vi "beginPrepareKickoffEnemyPlayVSS.vi"(8 "error in (no error)":errorcluster, 10 "Game in":refnum<class "Game.lvclass">, 11 "PrepareKickoffEnemyPlayVSS in":refnum<class "PrepareKickoffEnemyPlayVSS.lvclass">) -> (0 "error out":errorcluster, 2 "Boolean":bool, 3 "PrepareKickoffEnemyPlayVSS out":refnum<class "PrepareKickoffEnemyPlayVSS.lvclass">)   [LabVIEW 2020, in "PrepareKickoffEnemyPlayVSS.lvclass"]
uses:
  PrepareKickoffEnemyPlayVSS.lvclass
  Game_class/Game.lvclass
  Game_class/Game.lvclass/Game.ctl
  Game_class/Read Referee.vi
  Game_class/Read AllyRef.vi
  Ally_class/Ally.lvclass
  Referee_class/Referee.lvclass
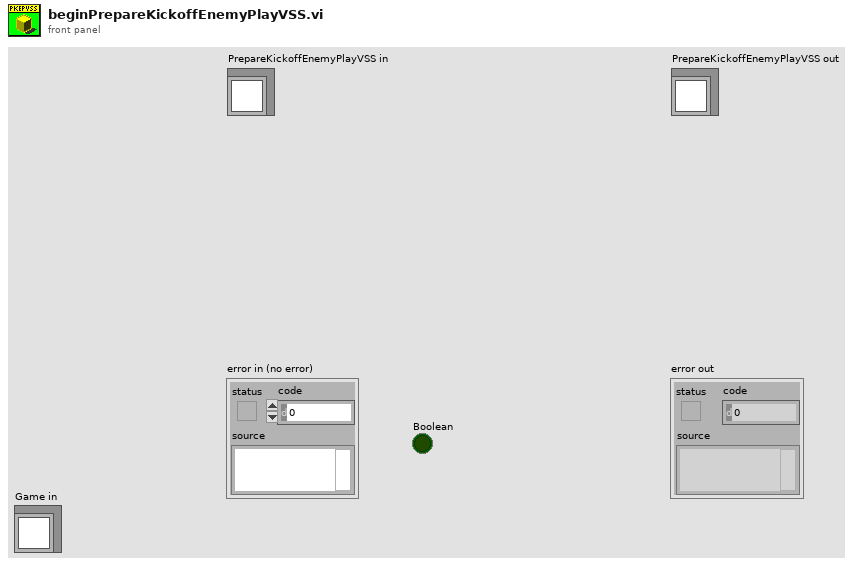
[diagram p1: front panel]
types:
  T1 = enum16{"AUTO", "GAME_ON", "STOP", "KICKOFF", "FREE_BALL", "GOAL_KICK", "PENALTY_KICK", "FREE_KICK"}
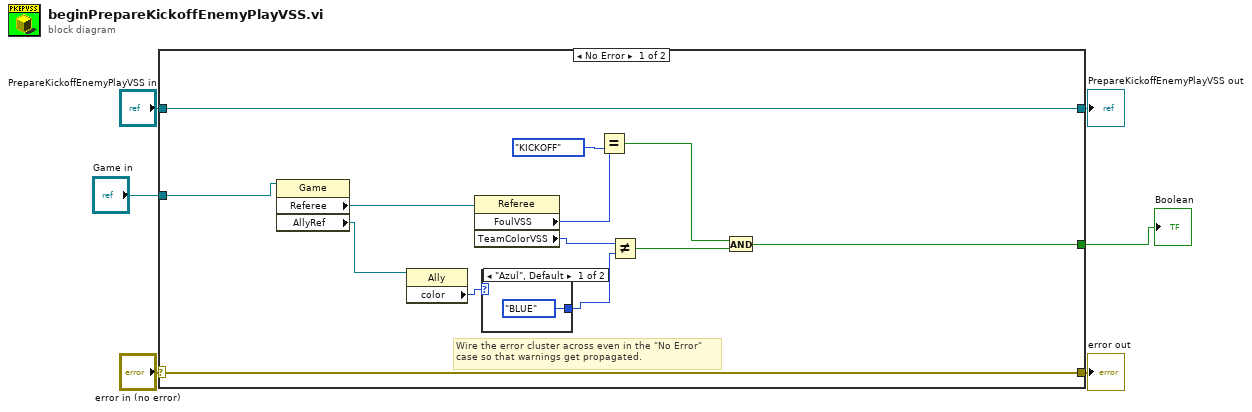
[diagram p0: block diagram]
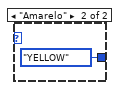
[diagram p2: hidden frame]
diagram:
  n1 = case shown="No Error" "error in (no error)" {
    selector: "error in (no error)" -> [w18 w23]
    tunnel: [w18 w23] -> w5
    tunnel: [w19 w22] -> w3
    tunnel: "PrepareKickoffEnemyPlayVSS in" -> [w19 w22]
    tunnel: "Game in" -> [w8 _]
    tunnel: [w7 _] -> w1
    frame No Error {
      # "Wire the error cluster across even in the \"No Error\"\ncase so that warnings get propagated."
      n2 = property class="Game"(reference=w8) -> ("Referee"=w17:refnum<class "Referee.lvclass">, "AllyRef"=w11:refnum<class "Ally.lvclass">)  [unwired: 1 in, 2 out]
      n3 = property class="Ally"(reference=w11) -> ("color"=w10:enum16{"Azul", "Amarelo"})  [unwired: 1 in, 2 out]
      n4 = property class="Referee"(reference=w17) -> ("FoulVSS"=w16:T1, "TeamColorVSS"=w13:enum16{"NONE", "YELLOW", "BLUE"})  [unwired: 1 in, 2 out]
      n5 = case shown="\"Azul\", Default" w10 {
        tunnel: [enum16{"NONE", "YELLOW", "BLUE"}."BLUE" ("TeamColorVSS") enum16{"NONE", "YELLOW", "BLUE"}."YELLOW" ("TeamColorVSS")] -> w9
        frame "Azul", Default {
        }
        frame "Amarelo" {
        }
      }
      n6 = Equal?(x=w16, y=T1."KICKOFF" ("FoulVSS")) -> (x = y?=w14:bool)
      n7 = Not Equal?(x=w13, y=w9) -> (x != y?=w12:bool)
      n8 = And(x=w14, y=w12) -> (x .and. y?=w7:bool)
    }
    frame Error {
    }
  }
  "error out" <- w5
  "PrepareKickoffEnemyPlayVSS out" <- w3
  "Boolean" <- w1
